vi "Cache.DUT.Find.vi"(6 "FileName Filter (empty: all)":string, 8 "error in (no error)":errorcluster, 9 "Size":i32, 10 "Page in":i32, 11 "Ref in use (empty: all)":string) -> (0 "error out":errorcluster, 1 "Pages":i32, 2 "Page out":i32, 3 "Products":string[](array[string]), 5 "Files":path[](array[path]), 7 "ModifyTS":timestamp[](array[timestamp]))   [LabVIEW 2016]
uses:
  Global/ApplicationGlobal.vi
panel:
  out "DELAY":u32
  out "Numeric":i32
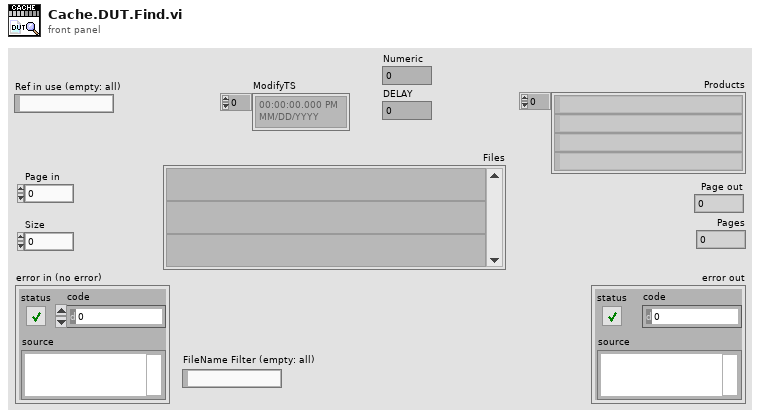
[diagram p1: front panel]
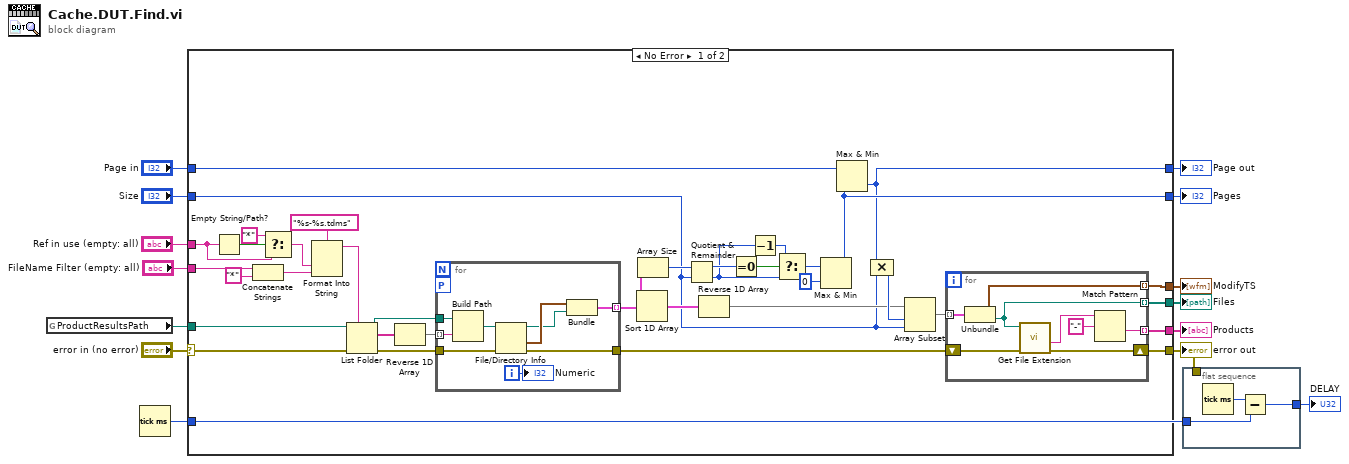
[diagram p0: block diagram]
diagram:
  n1 = global read "ApplicationGlobal.vi" "ProductResultsPath"() -> (w13:path)
  n2 = Tick Count (ms)() -> (millisecond timer value=w4:u32)
  n3 = case shown="No Error" "error in (no error)" {
    selector: "error in (no error)" -> [w50 w70]
    tunnel: [w15 w70] -> w5
    tunnel: w13 -> [w49 _]
    tunnel: "Ref in use (empty: all)" -> [w20 _]
    tunnel: [w32 _] -> w1
    tunnel: [w31 _] -> w2
    tunnel: "Size" -> [w27 w69]
    tunnel: "Page in" -> [w30 w68]
    tunnel: [w29 w69] -> w9
    tunnel: [w28 w68] -> w8
    tunnel: [w26 _] -> w7
    tunnel: "FileName Filter (empty: all)" -> [w18 _]
    tunnel: w4 -> [_ _]
    frame No Error {
      n4 = Empty String/Path?(string/path=w20) -> (empty?=w25:bool)
      n5 = Concatenate Strings(w18, "*" ("pattern")) -> (w19:string)
      n6 = Select(t="*" ("pattern"), s=w25, f=w20) -> (s? t:f=w21:string)
      n7 = Format Into String(format string="%s-%s.tdms", w21, w19) -> (resulting string=w22:string)  [unwired: 2 in, 1 out]
      n8 = List Folder(path=w49, pattern=w22, error in=w50) -> (path out=w46:path, filenames=w45:string[], error out=w47:errorcluster)  [unwired: 1 in, 1 out]
      n9 = Reverse 1D Array(array=w45) -> (reversed array=w48:string[])
      n10 = for {
        tunnel: w48 -> [w59] mode=indexing
        tunnel: w46 -> [w58]
        tunnel: [w56] -> w35 mode=indexing
        tunnel: w47 -> [w52]
        tunnel: [w57] -> w16
        workers-P: _ -> [_]
        i -> [w54]
        n11 = Build Path(base path=w58, name or relative path=w59) -> (appended path=w53:path)
        n12 = File/Directory Info(path=w53, error in=w52) -> (path out=w51:path, last mod=w55:timestamp, error out=w57:errorcluster)  [unwired: 4 out]
        n13 = Bundle("last mod"=w55, "path out"=w51) -> (w56:cluster{"last mod":timestamp, "path out":path})  [unwired: 1 in]
        "Numeric" <- w54
      }
      n14 = Sort 1D Array(array=w35) -> (sorted array=w44:cluster{"last mod":timestamp, "path out":path}[])
      n15 = Array Size(array=w35) -> (size(s)=w37:i32)
      n16 = Quotient & Remainder(x=w37, y=w27) -> (x-y*floor(x/y)=w42:i32, floor(x/y)=w40:i32)
      n17 = Reverse 1D Array(array=w44) -> (reversed array=w34:cluster{"last mod":timestamp, "path out":path}[])
      n18 = Equal To 0?(x=w42) -> (x = 0?=w41:bool)
      n19 = Decrement(x=w40) -> (x-1=w39:i32)
      n20 = Select(t=w39, s=w41, f=w40) -> (s? t:f=w38:i32)
      n21 = Max & Min(x=w38, y=0) -> (max(x,y)=w29:i32)  [unwired: 1 out]
      n22 = Max & Min(x=w30, y=w29) -> (min(x,y)=w28:i32)  [unwired: 1 out]
      n23 = Compound Arithmetic op=MULTIPLY(w28, w27) -> (w36:i32)
      n24 = Array Subset(array=w34, index=w36, length=w27) -> (w33:cluster{"last mod":timestamp, "path out":path}[])
      n25 = for {
        tunnel: w33 -> [w67] mode=indexing
        tunnel: [w60] -> w32 mode=indexing
        tunnel: [w64] -> w31 mode=indexing
        tunnel: [w66] -> w26 mode=indexing
        shift-right: [w63] -> w15
        shift-left: w16 -> [w65]
        n26 = Unbundle(w67) -> ("last mod"=w66:timestamp, "path out"=w64:path)
        n27 = call <vilib>:"Get File Extension.vi"("error in (no error)"=w65, "file"=w64) -> ("error out"=w63:errorcluster, "filename without extension"=w61:string)  [unwired: 5 in, 3 out]
        n28 = Match Pattern(string=w61, regular expression="-") -> (after substring=w60:string)  [unwired: 1 in, 3 out]
      }
    }
    frame Error {
    }
  }
  "error out" <- w5
  "Files" <- w2
  "Products" <- w1
  "Page out" <- w8
  "Pages" <- w9
  "ModifyTS" <- w7
  n29 = flat-sequence {
    tunnel: w5 -> [_]
    tunnel: w4 -> [w73]
    tunnel: [w71] -> w3
    frame #0 {
      n30 = Tick Count (ms)() -> (millisecond timer value=w72:u32)
      n31 = Subtract(x=w72, y=w73) -> (x-y=w71:u32)
    }
  }
  "DELAY" <- w3
